vi "Result Calculation.vi"(6 "shifting":bool=TRUE, 8 "Freq Response Limit":cluster{"Freq":dbl, "Upper":dbl, "Lower":dbl}[](array[cluster]), 9 "dB Reference":dbl=84.0, 10 "Frequency List":T1(array[cluster]), 11 "Fundamental-Response":T2(graph) caption="Fundamental-Response Mic1") -> (2 "Sensitivity Frequency (Hz)":dbl, 3 "Sensitivity (dBSPL)":dbl, 5 "Processed Freq Response":T2(graph) caption="Fundamental-Response Mic1", 7 "ProcessedFrequencyResponse":dbl[](array[numeric]))   [LabVIEW 2018]
panel:
  # "Result Calculation"
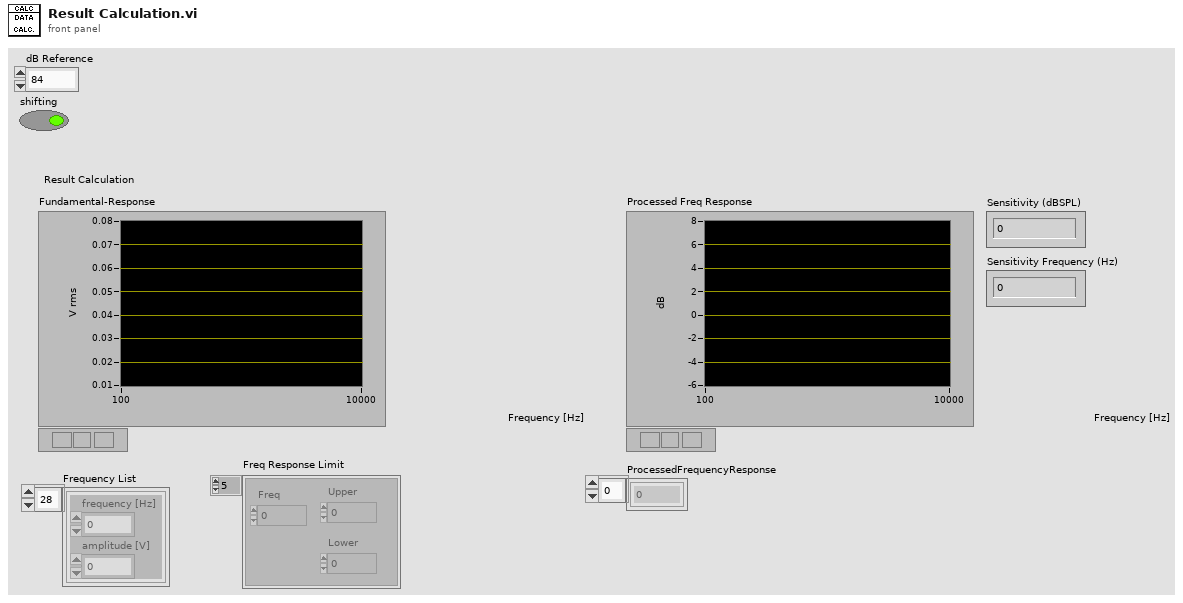
[diagram p1: front panel]
types:
  T1 = cluster{"frequency [Hz]":dbl, "amplitude [V]":dbl}[]
  T2 = cluster{"frequency [Hz]":dbl[], "amplitude":dbl[]}
  T3 = cluster{"frequency [Hz]":dbl[], "ProcessedFrequencyResponse":dbl[]}
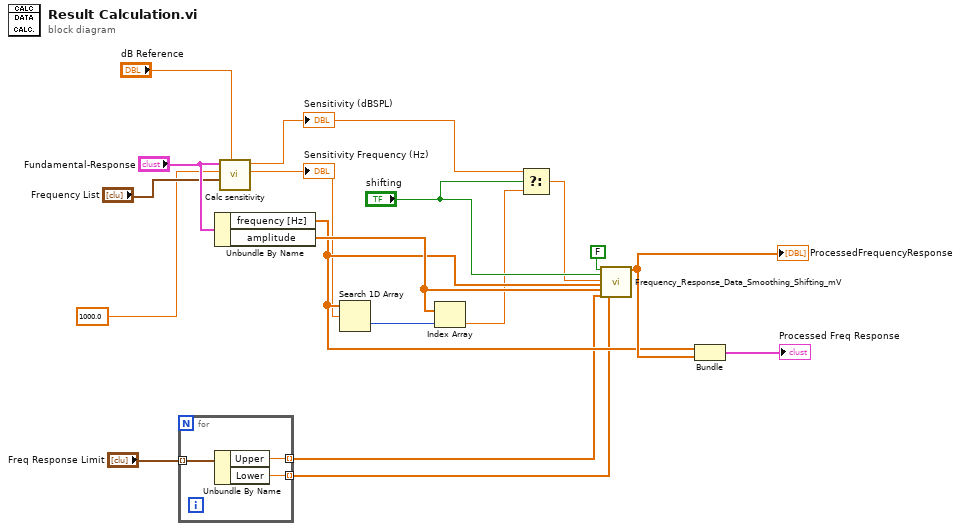
[diagram p0: block diagram]
diagram:
  n1 = for {
    tunnel: "Freq Response Limit" -> [w21] mode=indexing
    tunnel: [w20] -> w7 mode=indexing
    tunnel: [w19] -> w8 mode=indexing
    n2 = Unbundle By Name(w21) -> ("Upper"=w20:dbl, "Lower"=w19:dbl)
  }
  n3 = Unbundle By Name("Fundamental-Response") -> ("frequency [Hz]"=w12:dbl[], "amplitude"=w18:dbl[])
  n4 = call "Calc sensitivity.vi"("dB Reference"="dB Reference", "Frequency list Adjusted"="Frequency List", "Frequency [Hz]"=1000.0 ("element"), "Fundamental Response"="Fundamental-Response") -> ("Sensitivity Frequency (Hz)"=w10:dbl, "Sensitivity (mV/Pa)"=w3:dbl)  [unwired: 5 in, 1 out]
  "Sensitivity (dBSPL)" <- w3
  "Sensitivity Frequency (Hz)" <- w10
  n5 = Search 1D Array(1D array=w12, element=w10) -> (index of element=w5:i32)  [unwired: 1 in]
  n6 = Index Array(array=w18, index=w5) -> (element=w2:dbl)
  n7 = Select(t=w3, s="shifting", f=w2) -> (s? t:f=w1:dbl)
  n8 = call "Frequency_Response_Data_Smoothing_Shifting_mV.vi"("smoothing"=FALSE, "curveShifting"="shifting", "Parameters.RefAmplitude"=w1, "Parameters.UUTResponseLevel.frequency"=w12, "Parameters.UUTResponseLevel.amplitude"=w18, "FG.FrequencyLists.FrequencyResponse_LimitHigh.amplitude"=w7, "FG.FrequencyLists.FrequencyResponse_LimitLow.amplitude"=w8) -> ("ProcessedFrequencyResponse"=w17:dbl[])  [unwired: 12 in]
  "ProcessedFrequencyResponse" <- w17
  n9 = Bundle("frequency [Hz]"=w12, "ProcessedFrequencyResponse"=w17) -> (→"Processed Freq Response":T3)  [unwired: 1 in]
